vi "Test_LogValueEvent_LogMultipleDBLTimeBool_MatchFormattoString.vi"(8 "error in (no error)":errorcluster, 11 "TestCase in":refnum<class "TestLogValue.lvclass">) -> (0 "error out":errorcluster, 3 "TestCase out":refnum<class "TestLogValue.lvclass">)   [LabVIEW 2019, in "TestLogValue.lvclass"]
uses:
  TestLogValue.lvclass
  Source/Composed Log/Types/Log Level.ctl
  Source/Composed Log/LoggerReference/LoggerReference.lvclass/LoggerReference.ctl
  Source/LVQueue Sink/LVQueue Sink.lvclass/LVQueue Sink.ctl
  272d61b2-f49c-486c-9daf-337ffb054b40.vi
  154dbc8a-62f5-4aa1-ad82-2a3c469f95b7.vi
  Source/Composed Log/LoggerReference/Return Aggregate Queues.vi
  Source/Composed Log/LoggerReference/Add Aggregate Log.vi
  272d61b2-f49c-486c-9daf-337ffb054b40.vi/a63b633c-2cba-434f-a675-fad9ad4035ad.vi
  154dbc8a-62f5-4aa1-ad82-2a3c469f95b7.vi/c3b6b971-86f5-472c-b913-59f015cfd4c5.vi
  Source/Composed Log/LoggerReference/Get Formatter.vi
  Source/Composed Log/LoggerReference/Get Valid Event Time.vi
  Source/Composed Log/LoggerReference/Log Event.vi
  Source/Composed Log/LoggerReference/Send Add Sink.vi
  Source/Composed Log/LoggerReference/Log.vi
  Source/Composed Log/LoggerReference/Remove Stale Logs.vi
  Source/LVQueue Sink/LVQueue Sink.lvclass
  C:/CS/Log/Source/Composed Log/Log Sink/Log Sink.lvclass
  Source/Composed Log/Application Logger/Launch Worker Loop.vi
  Source/Composed Log/LoggerReference/Initialize Logger Instance.vi
  Source/Composed Log/LoggerReference/Format Variant.vi
  Source/Composed Log/LoggerReference/LoggerReference.lvclass
  Source/Composed Log/IErrorFormat/IErrorFormat.lvclass
  Source/Composed Log/Log Sink/Log Sink.lvclass
  <vilib>/addons/_JKI Toolkits/VI Tester/TestCase.llb/TestCase.lvclass
  Source/Composed Log/Composed Log.lvlib
  C:/Program Files (x86)/National Instruments/LabVIEW 2019/vi.lib/addons/_JKI Toolkits/VI Tester/TestCase.llb/TestCase.lvclass
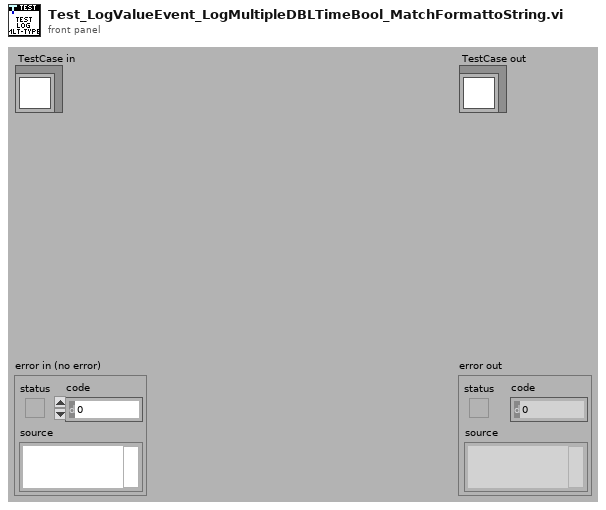
[diagram p1: front panel]
types:
  T1 = typedef "Composed Log.lvlib/Log Level.ctl" = enum16{"Debug", "Info", "Warning", "Error", "Critical"}
  T2 = typedef "Composed Log.lvlib/Log Packet.ctl" = cluster{"Data To Log":string, "Source":string, "Event Level":T1, "Event Time":timestamp}
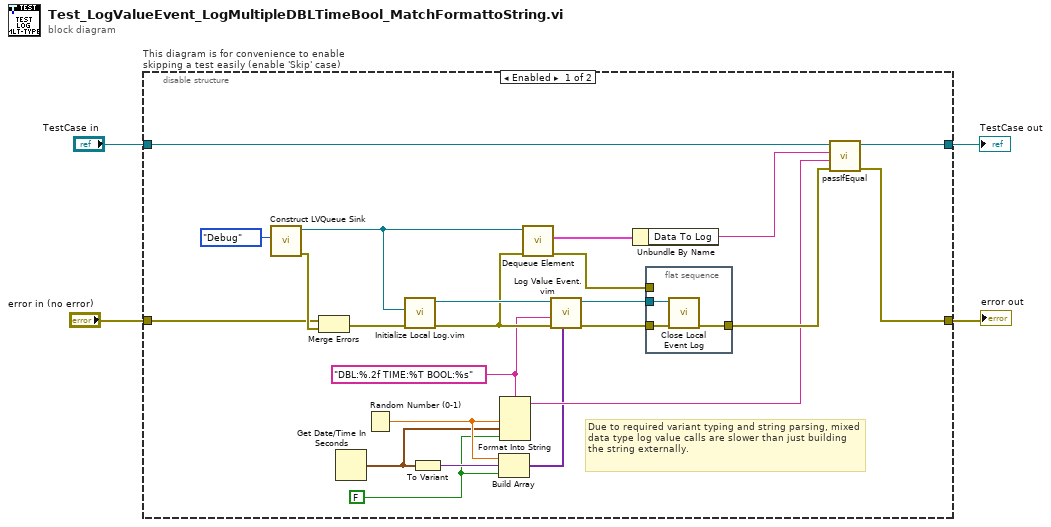
[diagram p0: block diagram]
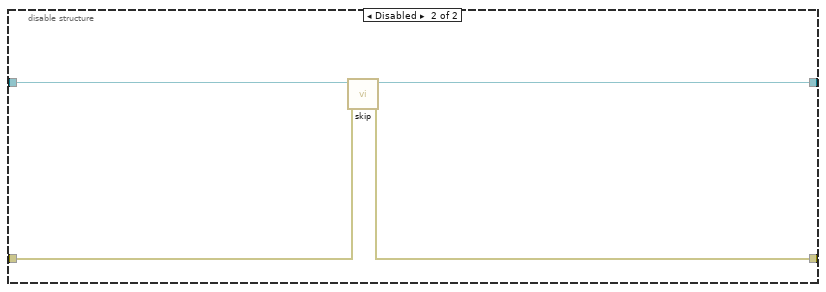
[diagram p2: hidden frame]
diagram:
  n1 = disable-structure "This diagram is for convenience to enable skipping a test easily (enable 'Skip' case)" shown="Enabled" {
    disable-tunnel: "TestCase in" -> [w21 w34]
    disable-tunnel: [w20 w32] -> w1
    disable-tunnel: [w18 w33] -> w3
    disable-tunnel: "error in (no error)" -> [w19 w31]
    frame Enabled {
      w5 = FALSE
      w13 = "DBL:%.2f TIME:%T BOOL:%s" ("Data To Log")
      # "Due to required variant typing and string parsing, mixed data type log value calls are slower than just building the string externally."
      n2 = call "Construct LVQueue Sink.vi"("LogLevel"=Log_Level."Debug") -> ("error out"=w24:errorcluster, "LVQueue Sink out"=w22:refnum<class "LVQueue Sink.lvclass">)  [unwired: 9 in]
      n3 = Merge Errors(w19, w24) -> (w23:errorcluster)
      n4 = Get Date/Time In Seconds() -> (seconds since 1Jan1904=w6:timestamp)
      n5 = Random Number (0-1)() -> (number: 0 to 1=w9:dbl)
      n6 = call "Initialize Local Log.vim"("error in (no error)"=w23, "Startup Sink(s)"=w22) -> ("error out"=w16:errorcluster, "Log Instance Reference"=w17:refnum<class "LoggerReference.lvclass">)  [unwired: 7 in, 1 out]
      n7 = To Variant(anything=w6) -> (Variant=w7:variant)
      n8 = Build Array(w9, w7, w5) -> (w8:variant[])
      n9 = Format Into String(format string=w13, w9, w6, w5) -> (resulting string=w11:string)  [unwired: 2 in, 1 out]
      n10 = call "Dequeue Element.vi"("error in (no error)"=w16, "LVQueue Sink in"=w22) -> ("error out"=w27:errorcluster, "Log Packet"=w25:T2)  [unwired: 6 in, 2 out]
      n11 = call "Log Value Event.vim"("Value(s)"=w8, "error in (no error)"=w16, "Log Message Format String"=w13, "LoggerReference in"=w17) -> ("error out"=w15:errorcluster, "LoggerReference out"=w14:refnum<class "LoggerReference.lvclass">)  [unwired: 6 in]
      n12 = Unbundle By Name(w25) -> ("Data To Log"=w12:string)
      n13 = flat-sequence {
        tunnel: [w29] -> w26
        tunnel: w15 -> [w30]
        tunnel: w27 -> [_]
        tunnel: w14 -> [w28]
        frame #0 {
          n14 = call "Close Local Event Log.vi"("error in (no error)"=w30, "Log Instance"=w28) -> ("error out"=w29:errorcluster)  [unwired: 9 in]
        }
      }
      n15 = call-dynamic "passIfEqual.vi"("error in (no error)"=w26, "y"=w11, "x"=w12, "TestCase in"=w21) -> ("error out"=w18:errorcluster, "TestCase out"=w20:refnum<class "TestLogValue.lvclass">)  [unwired: 6 in]
    }
    frame Disabled {
      # "skip test result while test is under development"
      n16 = call <vilib>:"skip.vi"("error in (no error)"=w31, "TestCase in"=w34) -> ("error out"=w33:errorcluster, "TestCase out"=w32:refnum<class "TestLogValue.lvclass">)  [unwired: 8 in]
    }
  }
  "error out" <- w3
  "TestCase out" <- w1
